vi "Lab 1 Parte 2 ex 1.vi"() -> ()   [LabVIEW 2020]
uses:
  <vilib>/MakerHub/LINX/Public/Peripherals/Digital/Digital Write 1 Chan.vi
  <vilib>/MakerHub/LINX/Public/Peripherals/Digital/Digital Write N Chans.vi
  <vilib>/MakerHub/LINX/Private/Local IO/LinxDigitalWrite.vi
  <vilib>/MakerHub/LINX/Public/Utilities/Check Channel.vi
  <vilib>/MakerHub/LINX/Public/Utilities/Open Serial.vi
  <vilib>/MakerHub/LINX/Public/Sensors/Motion/Servo/Servo Open One Channel.vi
  <vilib>/MakerHub/LINX/Public/Sensors/Motion/Servo/Servo Set Pulse Width One Channel.vi
  <vilib>/MakerHub/LINX/Private/Utilties/Generate Error.vi
  <vilib>/MakerHub/LINX/Public/Sensors/Motion/Servo/Servo Close One Channel.vi
  <vilib>/MakerHub/LINX/LMH-LINX.lvlib
  <vilib>/MakerHub/LINX/Public/Sensors/Motion/Servo/Servo.lvlib
panel:
  in  "STOP":bool
  out "High":bool=TRUE
  out "Medium":bool=TRUE
  out "Low":bool=TRUE
  in  "PWM Channel":u8
  in  "Pulse":dbl(slide) scale=0.0..2500.0
  in  "Serial Port":refnum<visa-resource-name>="N/A"
  out "Error Out":errorcluster
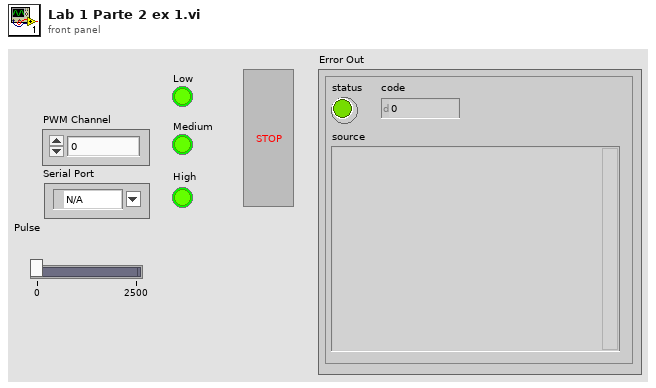
[diagram p1: front panel]
types:
  T1 = typedef "LMH-LINX.lvlib/LINX Ref.ctl" = cluster{"IO":T2, "Interface":T3, "LINX Device Config":T4}
  T2 = typedef "LMH-LINX.lvlib/Platform.ctl" = enum16{"Remote", "Local"}
  T3 = typedef "LMH-LINX.lvlib/Interface.ctl" = enum16{"Serial", "TCP"}
  T4 = typedef "LMH-LINX.lvlib/Device.lvlib/LINX Device Config.ctl" = cluster{"Interface":T3, "COM Port":refnum<visa-resource-name>, "TCP Configuration":T5, "Device Family":u8, "Device ID":u8, "Device Name":string, "TCP Ref":refnum<k5>, "Channels":T6}
  T5 = typedef "LMH-LINX.lvlib/Device.lvlib/TCP Config.ctl" = cluster{"IP Address":string, "Port":u16}
  T6 = typedef "LMH-LINX.lvlib/Channels.ctl" = cluster{"DI":u8[], "DO":u8[], "AI":u8[], "AO":u8[], "PWM":u8[], "QE":u8[], "UART":u8[], "I2C 2":u8[], "SPI":u8[], "CAN":u8[], "Servo":u8[], "AI Ref (V)":dbl, "AI Resolution (Bits)":u8, "AO Ref (V)":dbl, "AO Resolution (Bits)":u8}
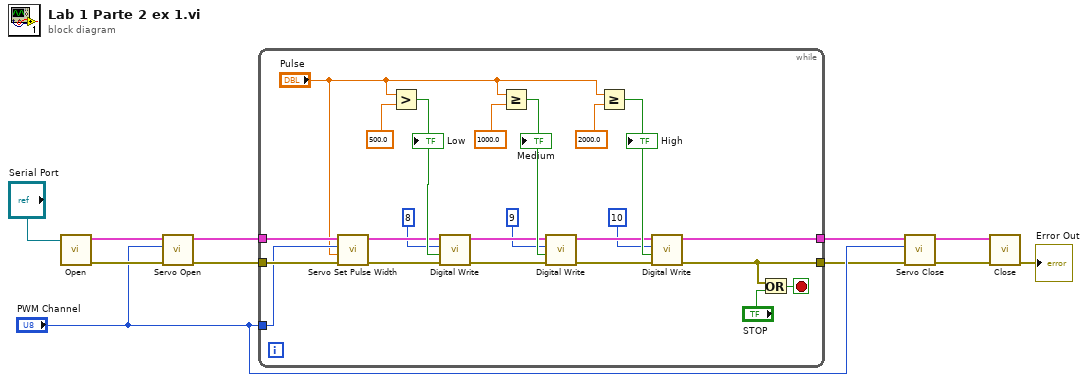
[diagram p0: block diagram]
diagram:
  n1 = call-poly <vilib>:"Open.vi"("Serial Port"="Serial Port") -> ("Error Out"=w8:errorcluster, "LINX Resource"=w9:T1)  [unwired: 8 in, 1 out]
  n2 = call-poly <vilib>:"Servo Open.vi"("Error In"=w8, "Servo Channel"="PWM Channel", "LINX Resource"=w9) -> ("Error Out"=w6:errorcluster, "LINX Resource"=w7:T1)  [unwired: 7 in]
  n3 = while {
    tunnel: [w26] -> w4
    tunnel: [w25] -> w3
    tunnel: "PWM Channel" -> [w20]
    tunnel: w7 -> [w24]
    tunnel: w6 -> [w21]
    stop <- w34 stop-if-true
    n4 = call-poly <vilib>:"Servo Set Pulse Width.vi"("Error In"=w21, "Pulse Width (uS)"="Pulse", "Servo Channel"=w20, "LINX Resource"=w24) -> ("Error Out"=w22:errorcluster, "LINX Resource"=w23:T1)  [unwired: 6 in]
    n5 = Greater?(x="Pulse", y=500.0 ("x")) -> (0:w33:bool)
    "Low" <- w33
    n6 = call-poly <vilib>:"Digital Write.vi"("Error In"=w22, "Output Value"=w33, "DO Channel"=8, "LINX Resource"=w23) -> ("Error Out"=w13:errorcluster, "LINX Resource"=w18:T1)  [unwired: 6 in]
    n7 = Greater Or Equal?(x="Pulse", y=1000.0 ("x")) -> (x >= y?=w27:bool)
    "Medium" <- w27
    n8 = call-poly <vilib>:"Digital Write.vi"("Error In"=w13, "Output Value"=w27, "DO Channel"=9, "LINX Resource"=w18) -> ("Error Out"=w12:errorcluster, "LINX Resource"=w17:T1)  [unwired: 6 in]
    n9 = Greater Or Equal?(x="Pulse", y=2000.0 ("x")) -> (x >= y?=w30:bool)
    "High" <- w30
    n10 = call-poly <vilib>:"Digital Write.vi"("Error In"=w12, "Output Value"=w30, "DO Channel"=10, "LINX Resource"=w17) -> ("Error Out"=w25:errorcluster, "LINX Resource"=w26:T1)  [unwired: 6 in]
    n11 = Or(x=w25, y="STOP") -> (x .or. y?=w34:bool)
  }
  n12 = call-poly <vilib>:"Servo Close.vi"("Error In"=w3, "Servo Channel"="PWM Channel", "LINX Resource"=w4) -> ("Error Out"=w1:errorcluster, "LINX Resource"=w2:T1)  [unwired: 7 in]
  n13 = call <vilib>:"Close.vi"("Error In"=w1, "LINX Resource"=w2) -> ("Error Out"=→"Error Out":errorcluster)  [unwired: 9 in]
